vi "DAQ_Shutdown.vi"(8 "error in":errorcluster, 11 "task/channels in":refnum<k21>) -> (0 "error out":errorcluster)   [LabVIEW 2026]
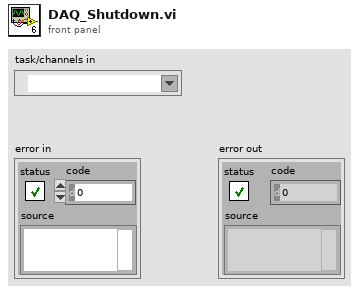
[diagram p1: front panel]
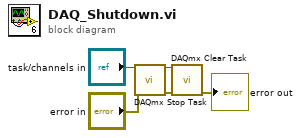
[diagram p0: block diagram]
diagram:
  n1 = call <vilib>:"DAQmx Stop Task.vi"("task/channels in"="task/channels in", "error in"="error in") -> ("task out"=w5:refnum<k21>, "error out"=w4:errorcluster)  [unwired: 12 in]
  n2 = call <vilib>:"DAQmx Clear Task.vi"("task in"=w5, "error in"=w4) -> ("error out"=→"error out":errorcluster)  [unwired: 13 in]
